vi "Read GUI Events.vi"(8 "Error In":errorcluster, 11 "BNT_SLTagMonitor in":refnum<class "BNT_SLTagMonitor.lvclass">) -> (0 "Error Out":errorcluster, 2 "GUI Events":T1, 3 "BNT_SLTagMonitor out":refnum<class "BNT_SLTagMonitor.lvclass">)   [LabVIEW 2019, in "BNT_SLTagMonitor.lvlib" / "BNT_SLTagMonitor.lvclass"]
doc: "Read GUI event references from attribute."
uses:
  BNT_SLTagMonitor.lvclass
  CSPP_Core/Messages/CSPP_PVUpdate Msg/CSPP_PVUpdate Msg.lvclass
  <vilib>/ActorFramework/Message Enqueuer/Message Enqueuer.lvclass
  <vilib>/Skyline/Tag/Wrapper/Wrapper_class/NI Skyline Tag.lvclass
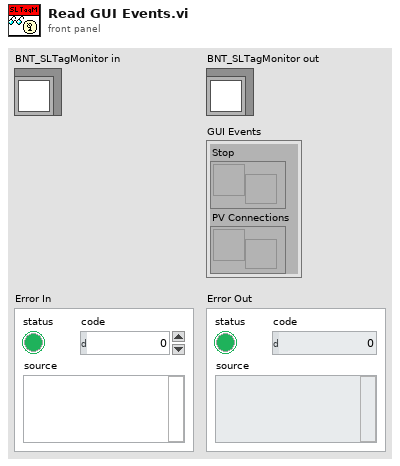
[diagram p1: front panel]
types:
  T1 = cluster{"Stop":refnum<user-event>, "PV Connections":refnum<user-event>}
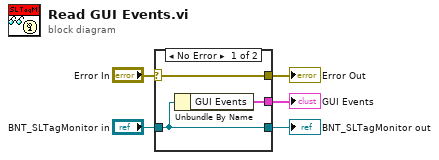
[diagram p0: block diagram]
diagram:
  n1 = case shown="No Error" "Error In" {
    selector: "Error In" -> [w8 w9]
    tunnel: [w8 w9] -> w2
    tunnel: [w7 w10] -> w4
    tunnel: "BNT_SLTagMonitor in" -> [w7 w10]
    tunnel: [w6 _] -> w3
    frame No Error {
      n2 = Unbundle By Name(w7) -> ("GUI Events"=w6:T1)
    }
    frame Error {
    }
  }
  "BNT_SLTagMonitor out" <- w4
  "GUI Events" <- w3
  "Error Out" <- w2
